vi "DecypherError.vi"(11 "Numeric":u8) -> (3 "error out":errorcluster)   [LabVIEW 2009]
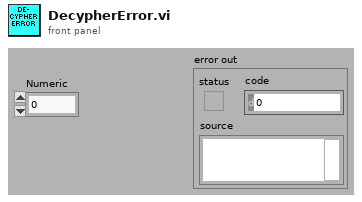
[diagram p1: front panel]
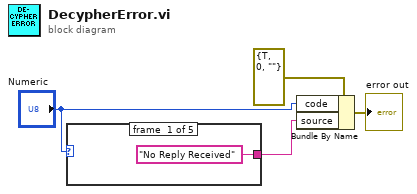
[diagram p0: block diagram]
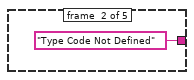
[diagram p2: hidden frame]
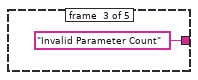
[diagram p3: hidden frame]
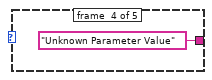
[diagram p4: hidden frame]
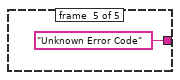
[diagram p5: hidden frame]
diagram:
  n1 = case shown="3" "Numeric" {
    tunnel: ["No Reply Received" ("source") "Type Code Not Defined" ("source") "Invalid Parameter Count" ("source") "Unknown Parameter Value" ("source") "Unknown Error Code" ("source")] -> w2
    frame #0 {
    }
    frame #1 {
    }
    frame #2 {
    }
    frame #3 {
    }
    frame #4 {
    }
  }
  n2 = Bundle By Name(cluster=errorcluster {"status"=TRUE, "code"=0, "source"=""} ("input cluster"), "code"="Numeric", "source"=w2) -> (→"error out":errorcluster)
